vi "Set Analog Replay.vi"(8 "error in (no error)":errorcluster, 9 "Analog Replay Data Options":T2={"Selected File"=path "", "Group"="", "Channel"="", "DataPlugin"="", "ReverseData"=FALSE, "FPGA memory size"=enum."16,384", "CycleAngle?"=enum."Crank angle", "Data Selection Method"=enum."Manual", "File start offset"=1, "Samples"=1, "Missing teeth location (degrees)"=1.0} {"Missing teeth location (degrees)" min=0.0; "Samples" min=1; "File start offset" min=0}, 10 "Analog Replay Settings":T1={"Name"="", "RIO Device Address"="", "DAC bipolar range (V)"=0.0001, "Voltage below min speed"=1.0, "Min speed (RPM)"=1.0, "Voltage at min speed"=1.0, "Max speed (RPM)"=1.0, "Voltage at max speed"=1.0, "ReverseNegate"=FALSE, "VOverride"=FALSE} {"Voltage at max speed" min=0.0 max=10.0; "Max speed (RPM)" min=1.0; "Voltage at min speed" min=0.0 max=10.0; "Min speed (RPM)" min=0.0; "Voltage below min speed" min=0.0 max=10.0; "DAC bipolar range (V)" min=0.0001}, 11 "Analog Replay in":refnum<k24>) -> (0 "error out":errorcluster, 3 "Analog Replay out":refnum<k24>)   [LabVIEW 2015, in "Engine Simulation Toolkit Scripting API.lvlib"]
uses:
  Engine Simulation Toolkit Scripting API.lvlib
  NationalInstruments.VeriStand.SystemDefinitionAPI
  Analog Replay Data Options.ctl
  System Explorer/FPGA Mem Size.ctl
  System Explorer/Position Reference.ctl
  System Explorer/Data Replay Data Selection Method.ctl
  Analog Replay Settings.ctl
  System Explorer/Engine Simulation Toolkit System Explorer.lvlib
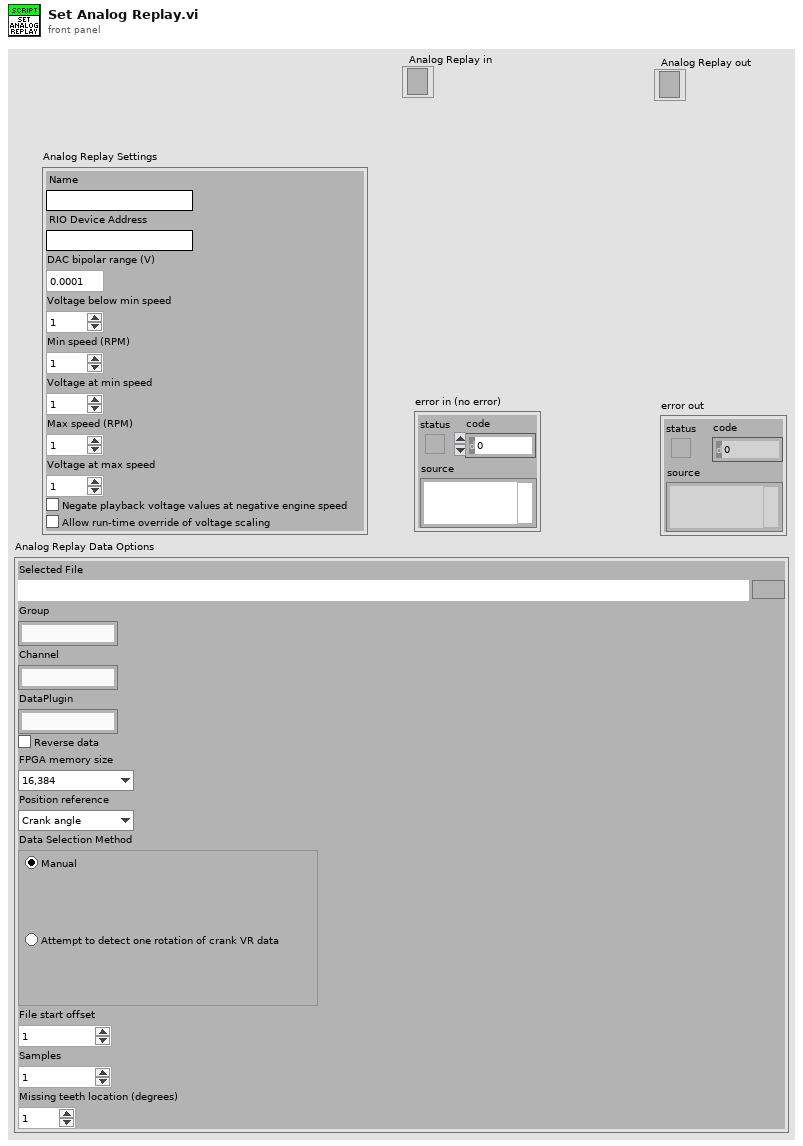
[diagram p1: front panel]
types:
  T1 = typedef "Engine Simulation Toolkit Scripting API.lvlib/Analog Replay Settings.ctl" = cluster{"Name":string, "RIO Device Address":string, "DAC bipolar range (V)":dbl, "Voltage below min speed":dbl, "Min speed (RPM)":dbl, "Voltage at min speed":dbl, "Max speed (RPM)":dbl, "Voltage at max speed":dbl, "ReverseNegate":bool, "VOverride":bool}
  T2 = typedef "Engine Simulation Toolkit Scripting API.lvlib/Analog Replay Data Options.ctl" = cluster{"Selected File":path, "Group":string, "Channel":string, "DataPlugin":string, "ReverseData":bool, "FPGA memory size":T3, "CycleAngle?":T4, "Data Selection Method":T5, "File start offset":i32, "Samples":i32, "Missing teeth location (degrees)":dbl}
  T3 = typedef "Engine Simulation Toolkit System Explorer.lvlib/FPGA Mem Size.ctl" = enum16{"65,536", "32,768", "16,384", "8,192", "4,096", "2,048", "1,024"}
  T4 = typedef "Engine Simulation Toolkit System Explorer.lvlib/Position Reference.ctl" = enum16{"Crank angle", "Cycle angle"}
  T5 = typedef "Engine Simulation Toolkit System Explorer.lvlib/Data Replay Data Selection Method.ctl" = enum32{"Manual", "AutoVRCrank"}
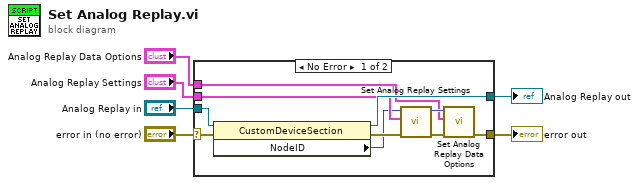
[diagram p0: block diagram]
diagram:
  n1 = case shown="No Error" "error in (no error)" {
    selector: "error in (no error)" -> [w15 w18]
    tunnel: [w7 w18] -> w6
    tunnel: "Analog Replay Data Options" -> [w8 _]
    tunnel: "Analog Replay in" -> [w16 w17]
    tunnel: "Analog Replay Settings" -> [w12 _]
    tunnel: [w13 w17] -> w1
    frame No Error {
      n2 = property class="CustomDeviceSection"(reference=w16, error in=w15) -> (reference out=w13:refnum<k24>, error out=w14:errorcluster, "NodeID"=w11:u64)
      n3 = call "Set Analog Replay Settings.vi"("error in (no error)"=w14, "Analog Replay Settings"=w12, "NodeID"=w11) -> ("error out"=w10:errorcluster, "NodeID"=w9:u64)  [unwired: 7 in]
      n4 = call "Set Analog Replay Data Options.vi"("error in (no error)"=w10, "Analog Replay Data Options"=w8, "NodeID"=w9) -> ("error out"=w7:errorcluster)  [unwired: 7 in, 1 out]
    }
    frame Error {
    }
  }
  "error out" <- w6
  "Analog Replay out" <- w1
